vi "Get_Sub_Collection.vi"(8 "error in (no error)":errorcluster caption="entrée d'erreur (pas d'erreur)", 11 "Firebase Benches en entrée":refnum<class "Firebase AssembledProducts.lvclass">) -> (0 "error out":errorcluster caption="sortie d'erreur", 3 "Firebase Benches en sortie":refnum<class "Firebase AssembledProducts.lvclass">)   [LabVIEW 2020, in "Library Instrument & Equipement.lvlib" / "Library FireBase.lvlib" / "Firebase AssembledProducts.lvclass"]
doc: "Return the documents present in the test collection for each DATA read with Get_Data\nPlease initialise the following values\n - Name BDD\n - Document of test sequence\n - API Key\n - Nb To Read"
uses:
  Firebase AssembledProducts.lvclass
  C:/Users/ngarcin/OneDrive - Altyor/Standard TB/Class/Firebase/Source/Firebase Driver/Firebase Driver.lvclass
  Firebase Altyor/Firebase Altyor.lvclass
  Firebase AssembledProducts.lvclass/Firebase AssembledProducts.ctl
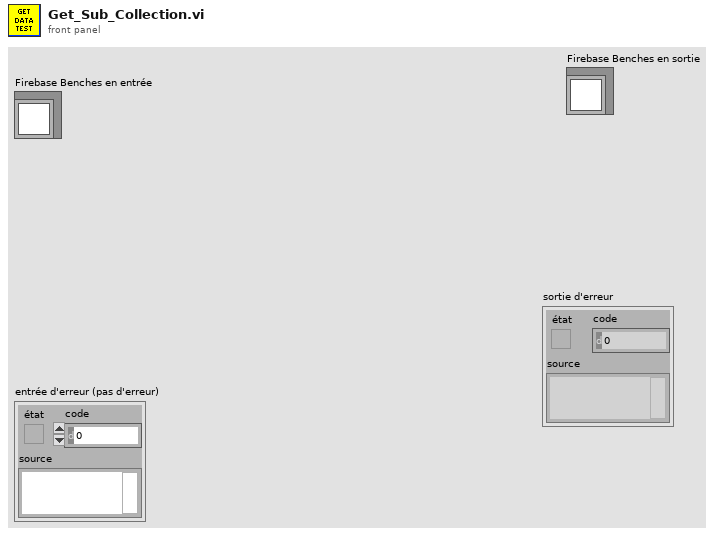
[diagram p1: front panel]
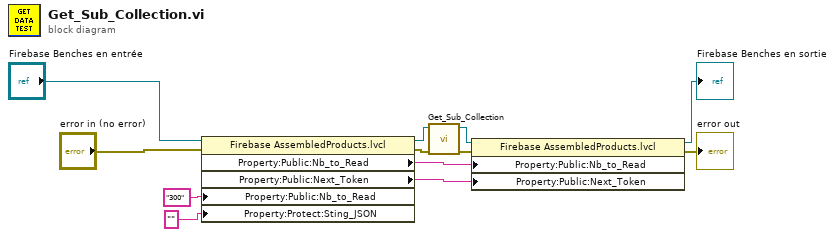
[diagram p0: block diagram]
diagram:
  n1 = property class="Firebase AssembledProducts.lvcl"(reference="Firebase Benches en entrée", error in="error in (no error)", "Property:Public:Nb_to_Read"="300" ("Nb_to_Read"), "Property:Protect:Sting_JSON"="" ("Next_Token")) -> (reference out=w8:refnum<class "Firebase AssembledProducts.lvclass">, error out=w9:errorcluster, "Property:Public:Nb_to_Read"=w5:string, "Property:Public:Next_Token"=w4:string)
  n2 = call-parent "Get_Sub_Collection.vi"("error in (no error)"=w9, "Firebase Altyor en entrée"=w8) -> ("error out"=w7:errorcluster, "Firebase Altyor en sortie"=w6:refnum<class "Firebase AssembledProducts.lvclass">)  [unwired: 8 in]
  n3 = property class="Firebase AssembledProducts.lvcl"(reference=w6, error in=w7, "Property:Public:Nb_to_Read"=w5, "Property:Public:Next_Token"=w4) -> (reference out=→"Firebase Benches en sortie":refnum<class "Firebase AssembledProducts.lvclass">, error out=→"error out":errorcluster)
